vi "synth_set (SubVI).vi"(5 "User Def. Wfm Name":string="RANDFREQ", 7 "wfm?":bool, 8 "error in (no error)":errorcluster, 9 "VISA session":refnum<visa-resource-name>, 11 "Tot Synth Arr":dbl[](array[numeric])) -> (0 "error out":errorcluster, 1 "dup VISA session":refnum<visa-resource-name>, 3 "Set synth?":bool)   [LabVIEW 2014]
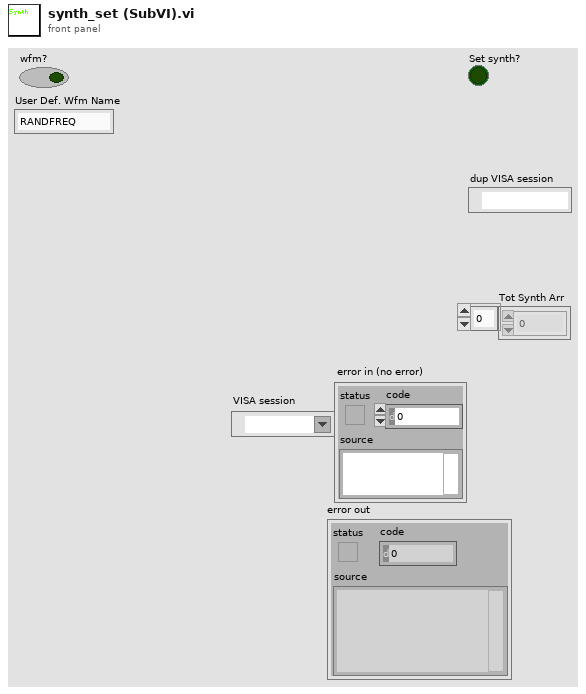
[diagram p1: front panel]
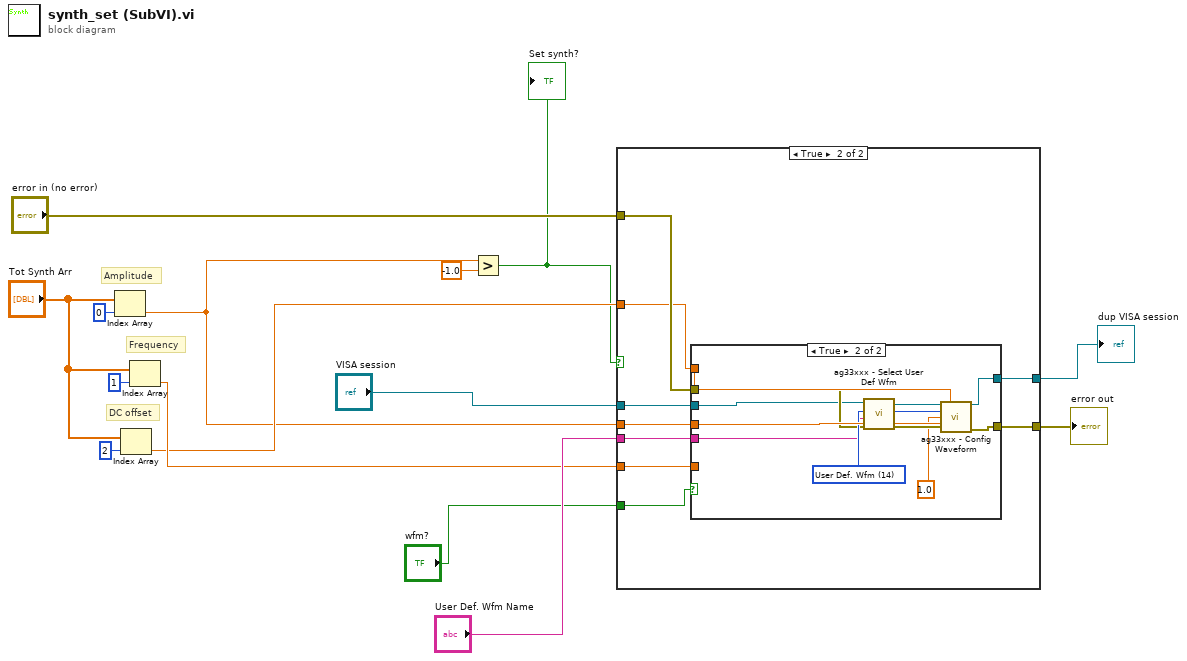
[diagram p0: block diagram]
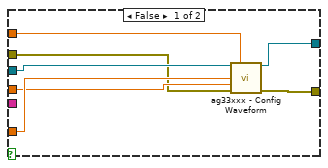
[diagram p3: hidden frame]
diagram:
  # "DC offset"
  # "Frequency"
  # "Amplitude"
  n1 = Index Array(array="Tot Synth Arr", index=0) -> (element=w5:dbl)
  n2 = Index Array(array="Tot Synth Arr", index=2) -> (element=w6:dbl)
  n3 = Index Array(array="Tot Synth Arr", index=1) -> (element=w9:dbl)
  n4 = Greater?(x=w5, y=-1.0) -> (0:w3:bool)
  "Set synth?" <- w3
  n5 = case shown="True" w3 {
    tunnel: "VISA session" -> [w16 w26]
    tunnel: "error in (no error)" -> [w17 w25]
    tunnel: "wfm?" -> [_ w24]
    tunnel: [w17 w23] -> w13
    tunnel: "User Def. Wfm Name" -> [_ w22]
    tunnel: w5 -> [_ w21]
    tunnel: w9 -> [_ w20]
    tunnel: w6 -> [_ w19]
    tunnel: [w16 w18] -> w2
    frame False {
    }
    frame True {
      n6 = case shown="True" w24 {
        tunnel: w26 -> [w29 w39]
        tunnel: w25 -> [w28 w40]
        tunnel: w19 -> [w33 w44]
        tunnel: w20 -> [w32 _]
        tunnel: w21 -> [w31 w43]
        tunnel: [w30 w41] -> w23
        tunnel: w22 -> [_ w36]
        tunnel: [w27 w34] -> w18
        frame False {
          n7 = call "ag33xxx - Config Waveform.vi"("VISA session"=w29, "Offset (0.00 V)"=w33, "Frequency (1000 Hz)"=w32, "Amplitude (0.1 Vpp)"=w31, "error in (no error)"=w28) -> ("dup VISA session"=w27:refnum<visa-resource-name>, "error out"=w30:errorcluster)  [unwired: 9 in]
        }
        frame True {
          w42 = u16 14 items=["DC"=0, "Sine"=1, "Square"=2, "Triangle"=3, "Ramp"=4, "Pulse"=6, "Noise"=7, "Sinc"=8, "Neg. Ramp"=9, "Exp. Rise"=10, "Exp. Fall"=11, "Cardiac"=12, "Volatile"=13, "User Def. Wfm"=14] ("Waveform Shape (1: Sine)")
          n8 = call "ag33xxx - Select User Def Wfm.vi"("error in (no error)"=w40, "User Def. Wfm Name"=w36, "VISA session"=w39) -> ("error out"=w37:errorcluster, "dup VISA session"=w38:refnum<visa-resource-name>)  [unwired: 7 in]
          n9 = call "ag33xxx - Config Waveform.vi"("VISA session"=w38, "Offset (0.00 V)"=w44, "Waveform Shape (1: Sine)"=w42, "Frequency (1000 Hz)"=1.0, "Amplitude (0.1 Vpp)"=w43, "error in (no error)"=w37) -> ("dup VISA session"=w34:refnum<visa-resource-name>, "error out"=w41:errorcluster)  [unwired: 8 in]
        }
      }
    }
  }
  "error out" <- w13
  "dup VISA session" <- w2
